vi "Hormiga_PBRead.vi"(8 "error in (no error)":errorcluster, 10 "Terminal":u8=13, 11 "VISA Refnum in":refnum<visa-resource-name>) -> (0 "error out":errorcluster, 2 "Returned Value":u16, 3 "VISA Refnum out":refnum<visa-resource-name>)   [LabVIEW 2016]
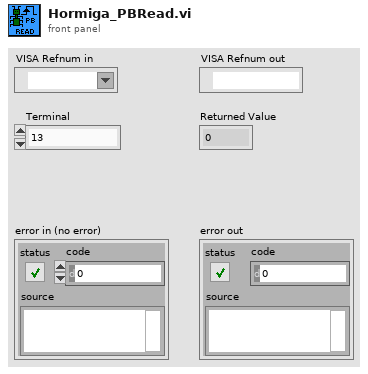
[diagram p1: front panel]
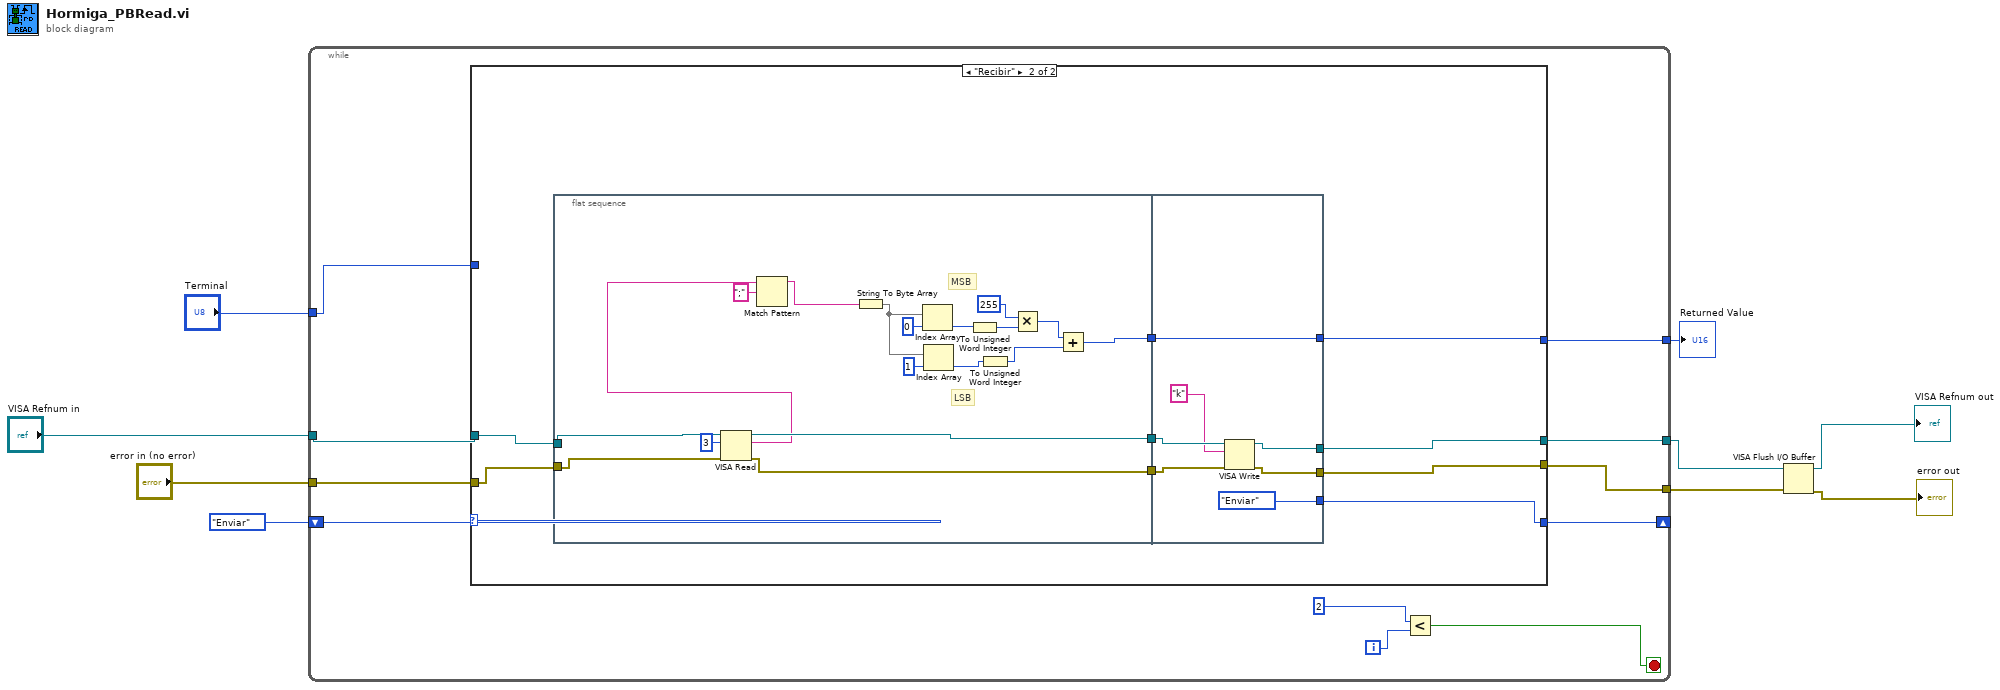
[diagram p0: block diagram]
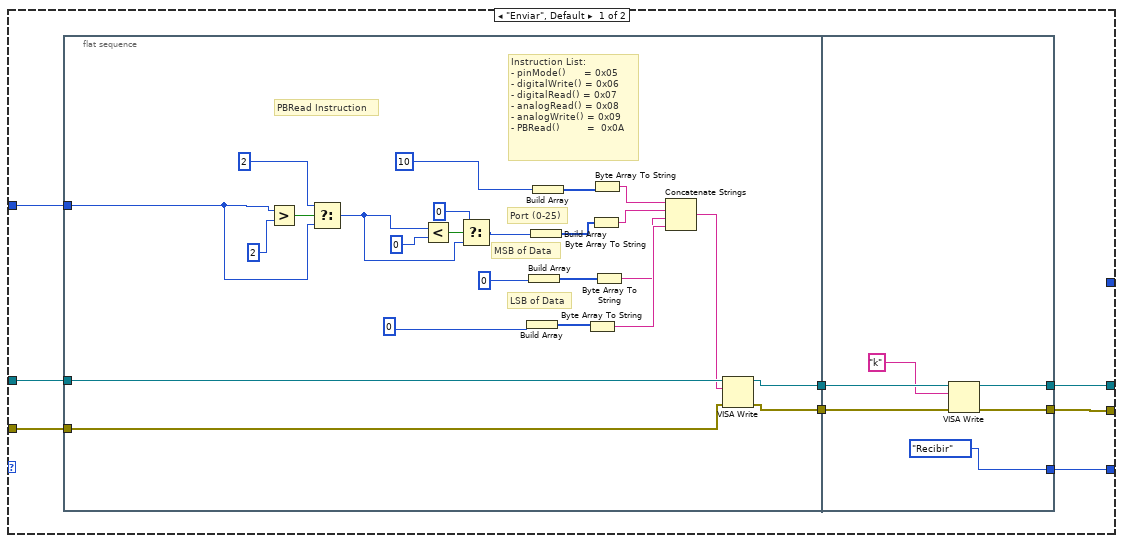
[diagram p2: hidden frame]
diagram:
  n1 = while {
    shift-right: [w15] -> _
    shift-left: enum16{"Enviar", "Recibir"}."Enviar" -> [w20]
    tunnel: "error in (no error)" -> [w19]
    tunnel: "VISA Refnum in" -> [w18]
    tunnel: [w17] -> w4
    tunnel: [w16] -> w3
    tunnel: "Terminal" -> [w11]
    tunnel: [w10] -> w9
    i -> [w13]
    stop <- w14 stop-if-true
    n2 = case shown="\"Recibir\"" w20 {
      tunnel: w19 -> [w28 w68]
      tunnel: w18 -> [w27 w67]
      tunnel: [w24 w64] -> w17
      tunnel: [w23 w63] -> w16
      tunnel: [w22 w62] -> w15
      tunnel: w11 -> [w21 _]
      tunnel: [_ w60] -> w10
      frame "Enviar", Default {
        n3 = flat-sequence {
          tunnel: w28 -> [w53]
          tunnel: w27 -> [w52]
          tunnel: [w51] -> w26
          tunnel: [w50] -> w25
          tunnel: w21 -> [w32]
          tunnel: w26 -> [w59]
          tunnel: w25 -> [w58]
          tunnel: [w56] -> w24
          tunnel: [w55] -> w23
          tunnel: [enum16{"Enviar", "Recibir"}."Recibir"] -> w22
          frame #0 {
            # "PBRead Instruction"
            # "Instruction List:\n- pinMode()      = 0x05\n- digitalWrite() = 0x06\n- digitalRead() = 0x07\n- analogRead() = 0x08\n- analogWrite() = 0x09\n- PBRead()         =  0x0A"
            # "LSB of Data"
            # "MSB of Data"
            # "Port (0-25)"
            n4 = Greater?(x=w32, y=u8 2) -> (0:w39:bool)
            n5 = Select(t=u8 2, s=w39, f=w32) -> (s? t:f=w34:u8)
            n6 = Less?(x=w34, y=u8 0) -> (x < y?=w36:bool)
            n7 = Select(t=u8 0, s=w36, f=w34) -> (s? t:f=w33:u8)
            n8 = Build Array(u8 0) -> (w45:u8[])
            n9 = Build Array(u8 0) -> (w46:u8[])
            n10 = Build Array(w33) -> (w47:u8[])
            n11 = Build Array(u8 10) -> (w48:u8[])
            n12 = Byte Array To String(unsigned byte array=w45) -> (string=w44:string)
            n13 = Byte Array To String(unsigned byte array=w47) -> (string=w42:string)
            n14 = Byte Array To String(unsigned byte array=w48) -> (string=w41:string)
            n15 = Byte Array To String(unsigned byte array=w46) -> (string=w43:string)
            n16 = Concatenate Strings(w41, w42, w43, w44) -> (w31:string)
            n17 = VISA Write(VISA resource name=w52, write buffer=w31, error in (no error)=w53) -> (VISA resource name out=w50:refnum<visa-resource-name>, error out=w51:errorcluster)  [unwired: 1 out]
          }
          frame #1 {
            n18 = VISA Write(VISA resource name=w58, write buffer="k", error in (no error)=w59) -> (VISA resource name out=w55:refnum<visa-resource-name>, error out=w56:errorcluster)  [unwired: 1 out]
          }
        }
      }
      frame "Recibir" {
        n19 = flat-sequence {
          tunnel: w68 -> [w78]
          tunnel: w67 -> [w77]
          tunnel: [w86] -> w66
          tunnel: [w85] -> w65
          tunnel: [w79] -> w61
          tunnel: w66 -> [w93]
          tunnel: w65 -> [w92]
          tunnel: [w90] -> w64
          tunnel: [w89] -> w63
          tunnel: [enum16{"Enviar", "Recibir"}."Enviar"] -> w62
          tunnel: w61 -> [w87]
          tunnel: [w87] -> w60
          frame #0 {
            # "MSB"
            # "LSB"
            n20 = VISA Read(VISA resource name=w77, byte count=u32 3, error in (no error)=w78) -> (VISA resource name out=w85:refnum<visa-resource-name>, read buffer=w75:string, error out=w86:errorcluster)  [unwired: 1 out]
            n21 = Match Pattern(string=w75, regular expression=";") -> (before substring=w73:string)  [unwired: 1 in, 3 out]
            n22 = String To Byte Array(string=w73) -> (unsigned byte array=w84:u8[])
            n23 = Index Array(array=w84, index=0) -> (element=w72:u8)
            n24 = Index Array(array=w84, index=1) -> (element=w70:u8)
            n25 = To Unsigned Word Integer(number=w72) -> (unsigned 16bit integer=w71:u16)
            n26 = To Unsigned Word Integer(number=w70) -> (unsigned 16bit integer=w69:u16)
            n27 = Multiply(x=u16 255, y=w71) -> (x*y=w81:u16)
            n28 = Add(x=w81, y=w69) -> (x+y=w79:u16)
          }
          frame #1 {
            n29 = VISA Write(VISA resource name=w92, write buffer="k", error in (no error)=w93) -> (VISA resource name out=w89:refnum<visa-resource-name>, error out=w90:errorcluster)  [unwired: 1 out]
          }
        }
      }
    }
    n30 = Less?(x=2, y=w13) -> (x < y?=w14:bool)
  }
  "Returned Value" <- w9
  n31 = VISA Flush I/O Buffer(VISA resource name=w3, error in (no error)=w4) -> (VISA resource name out=→"VISA Refnum out":refnum<visa-resource-name>, error out=→"error out":errorcluster)  [unwired: 1 in]
